vi "arduino_data_and_filters_subIV.vi"(7 "loop iteration number":i32, 8 "arduino 1-6 address and errors":T3, 11 "arduinos on?":bool) -> (0 "arduino 1-6 addresses and errors out":T2, 1 "arduino 1-6 data out":T1, 3 "arduinos on? output":bool)   [LabVIEW 2014]
uses:
  LabVIEW QCM code version 4 Working/(SubVI)2 2QCM.vi
  LabVIEW QCM code version 4 Working/(SubVI)1 3QCM.vi
  LabVIEW QCM code version 4 Working/(SubVI)2 3QCM.vi
  LabVIEW QCM code version 4 Working/(SubVI)1 4QCM.vi
  LabVIEW QCM code version 4 Working/(SubVI)2 4QCM.vi
  LabVIEW QCM code version 4 Working/(SubVI)1 5QCM.vi
  LabVIEW QCM code version 4 Working/(SubVI)2 5QCM.vi
  LabVIEW QCM code version 4 Working/(SubVI)1 6QCM.vi
  LabVIEW QCM code version 4 Working/(SubVI)2 6QCM.vi
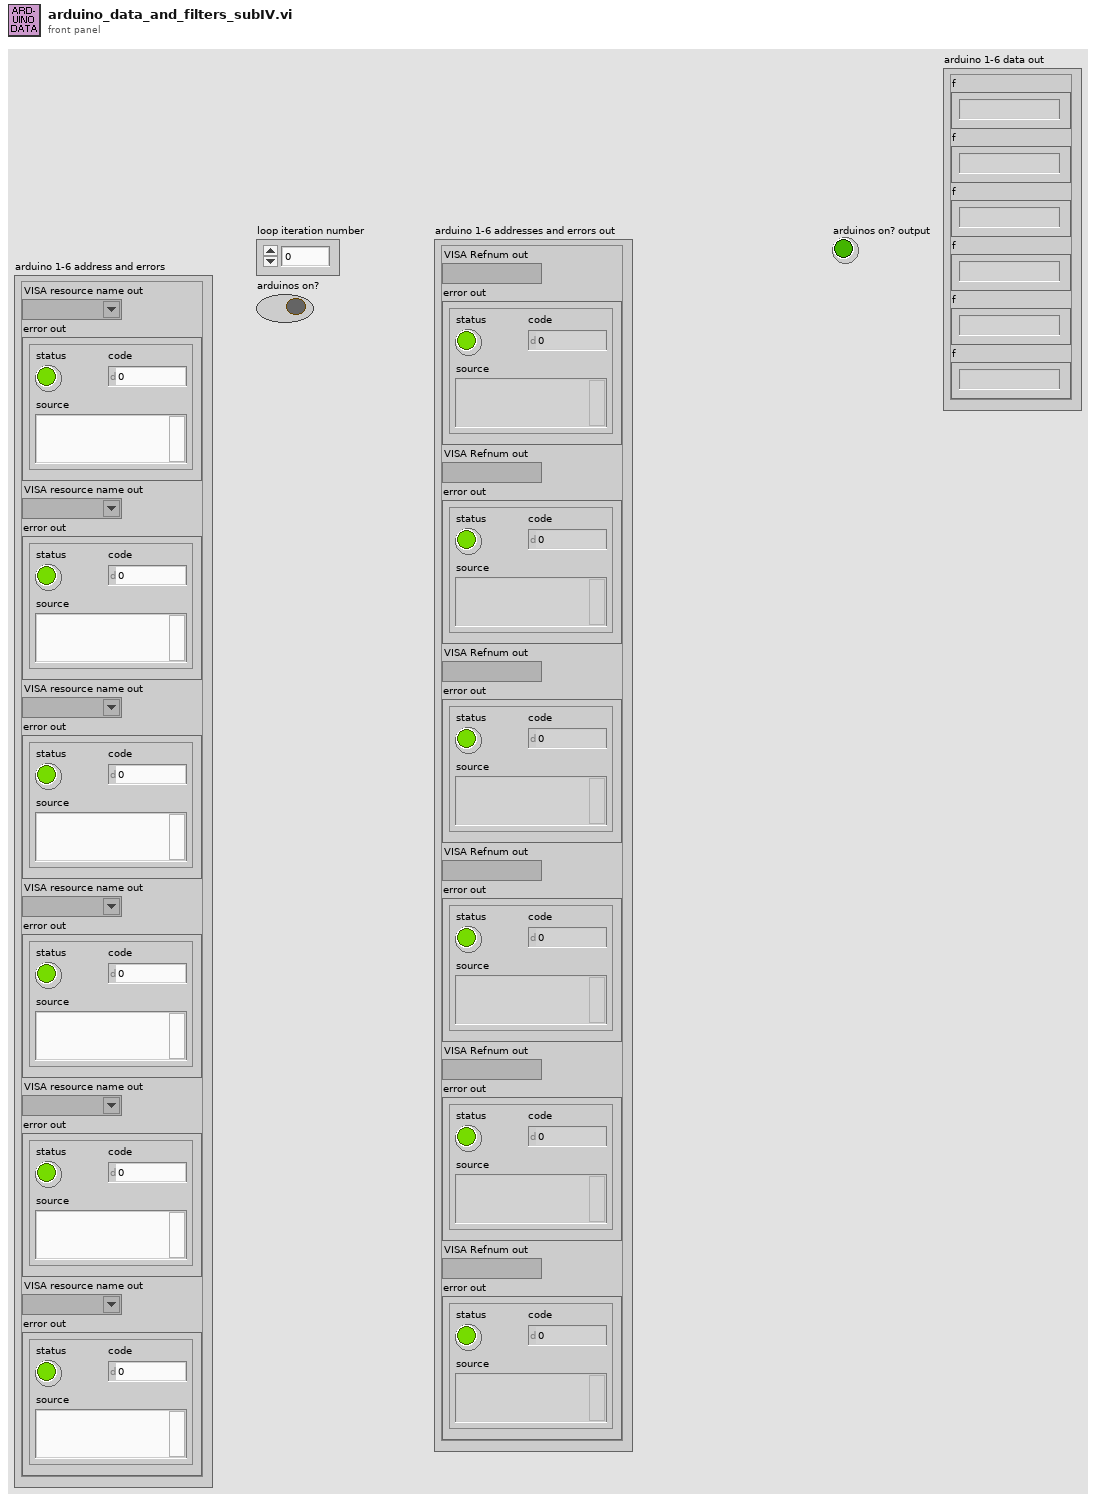
[diagram p1: front panel]
types:
  T1 = cluster{"f":string, "f":string, "f":string, "f":string, "f":string, "f":string}
  T2 = cluster{"VISA Refnum out":refnum<visa-resource-name>, "error out":errorcluster, "VISA Refnum out":refnum<visa-resource-name>, "error out":errorcluster, "VISA Refnum out":refnum<visa-resource-name>, "error out":errorcluster, "VISA Refnum out":refnum<visa-resource-name>, "error out":errorcluster, "VISA Refnum out":refnum<visa-resource-name>, "error out":errorcluster, "VISA Refnum out":refnum<visa-resource-name>, "error out":errorcluster}
  T3 = cluster{"VISA resource name out":refnum<visa-resource-name>, "error out":errorcluster, "VISA resource name out":refnum<visa-resource-name>, "error out":errorcluster, "VISA resource name out":refnum<visa-resource-name>, "error out":errorcluster, "VISA resource name out":refnum<visa-resource-name>, "error out":errorcluster, "VISA resource name out":refnum<visa-resource-name>, "error out":errorcluster, "VISA resource name out":refnum<visa-resource-name>, "error out":errorcluster}
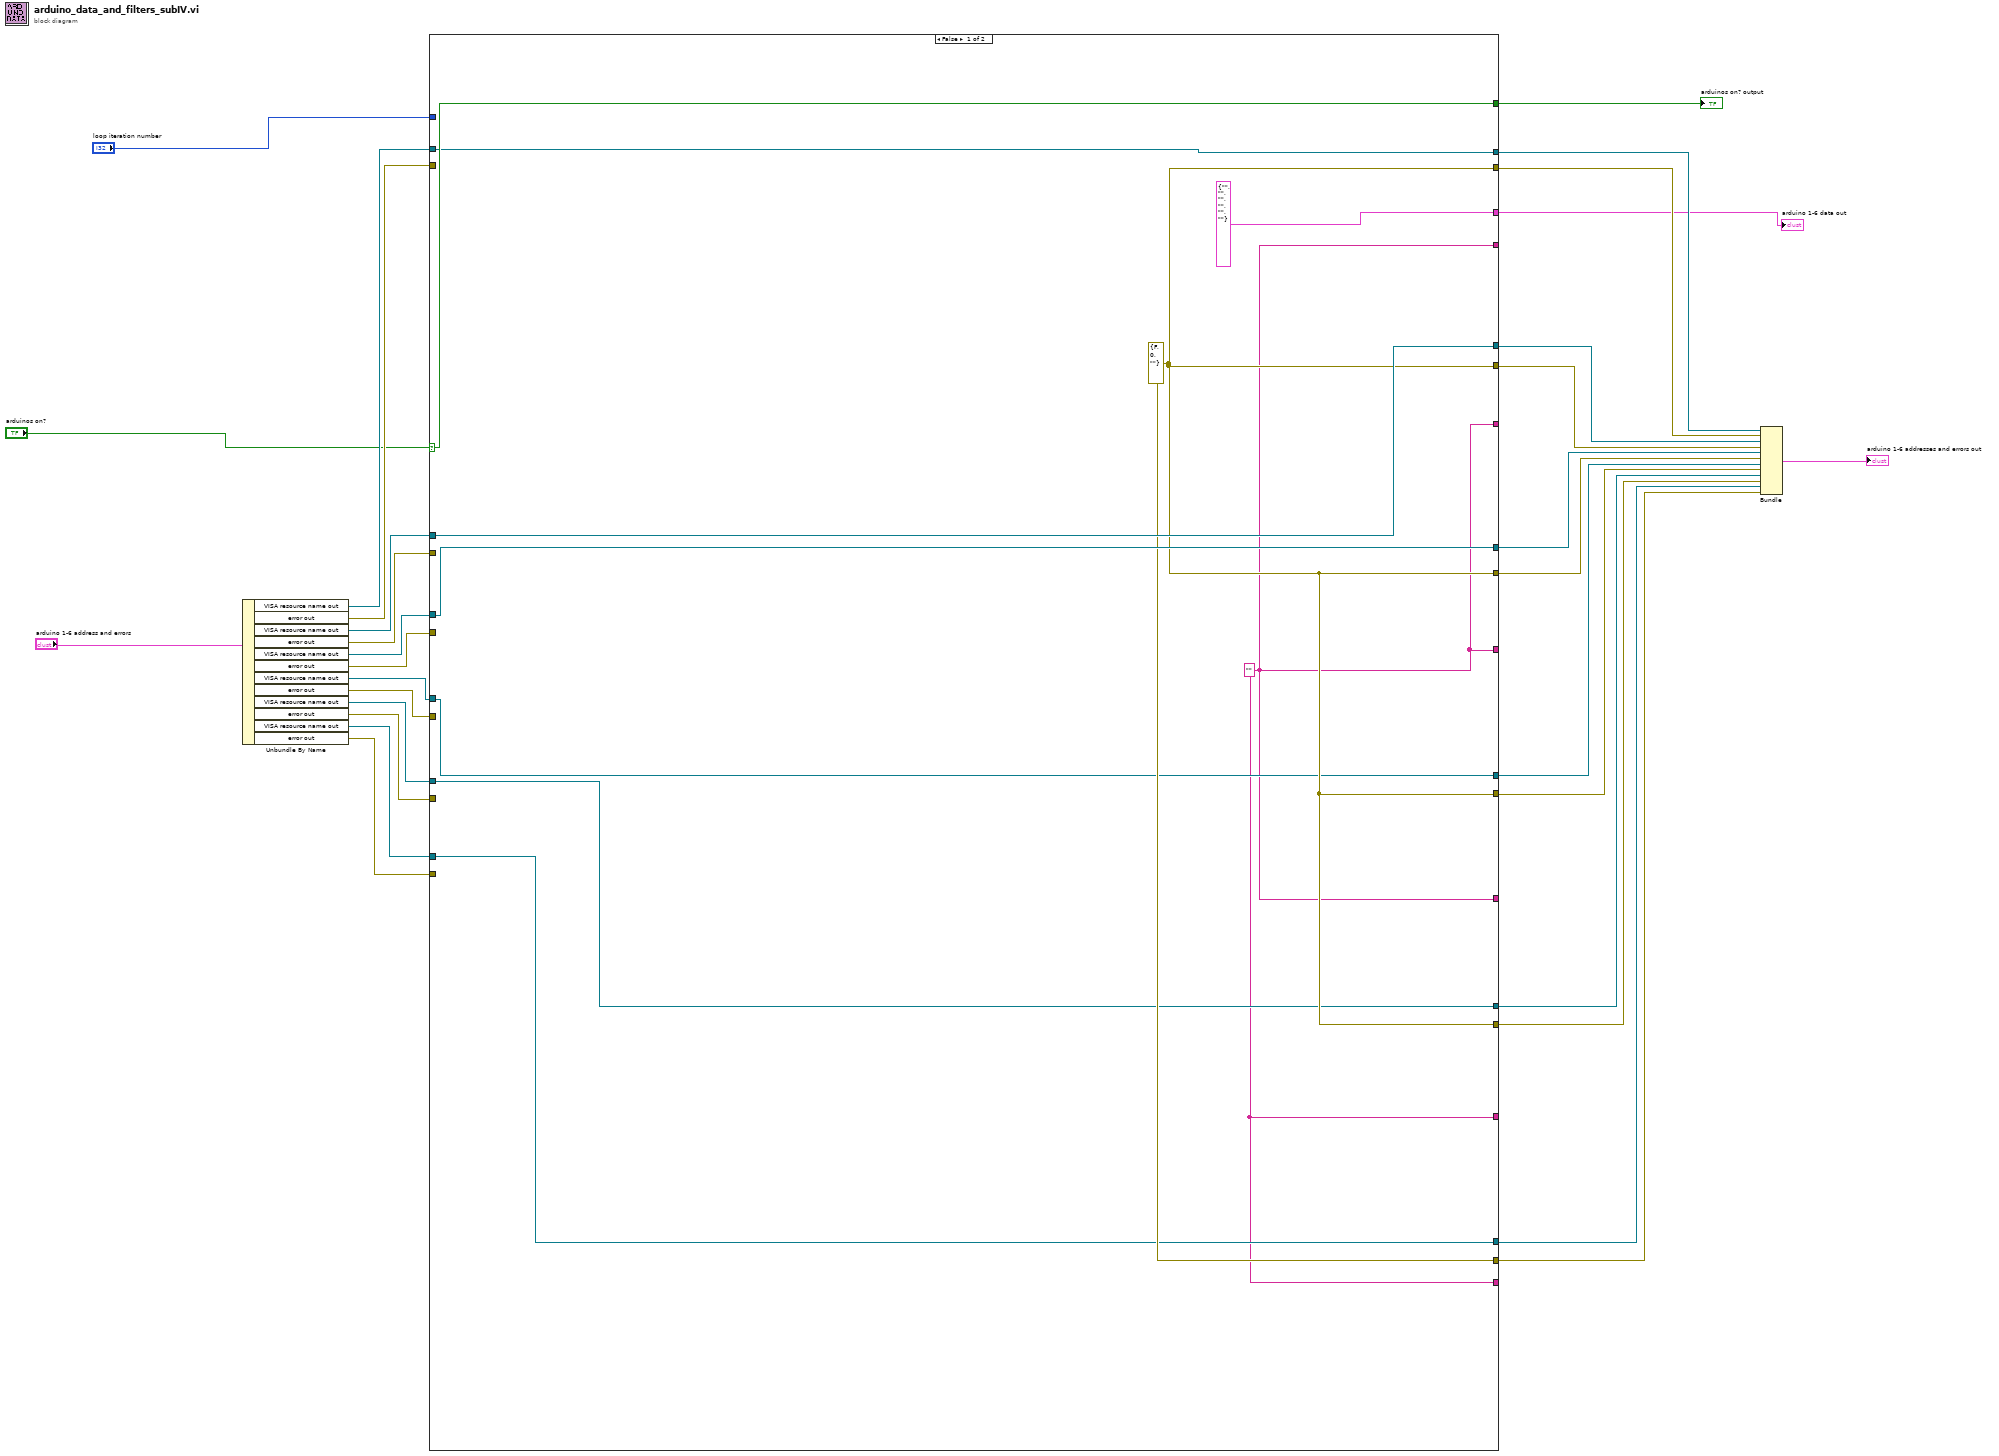
[diagram p0: block diagram]
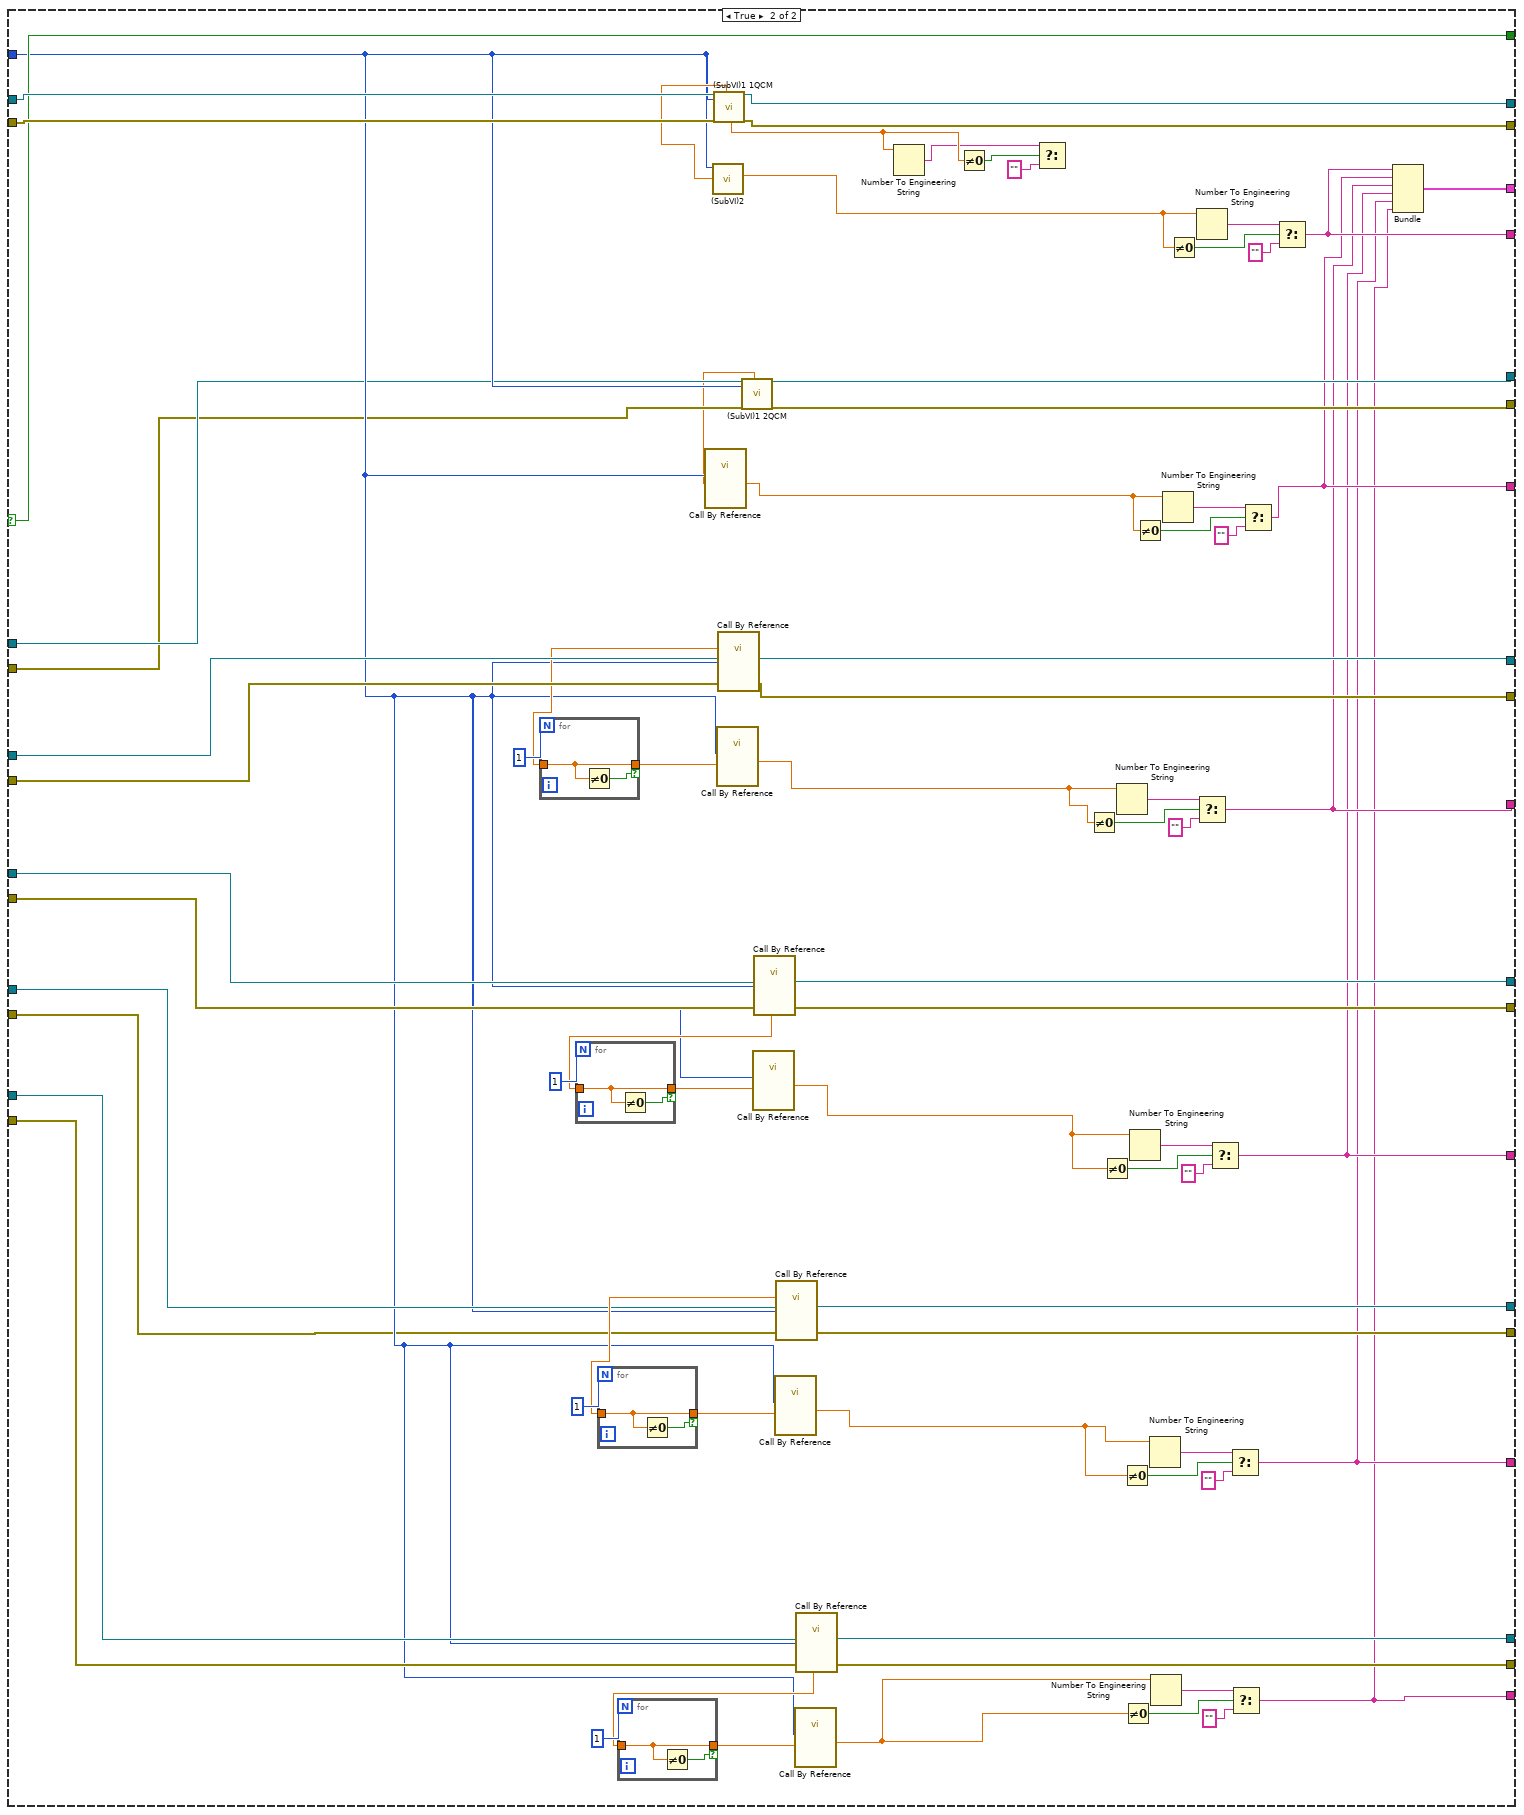
[diagram p2: hidden frame]
diagram:
  n1 = Unbundle By Name("arduino 1-6 address and errors") -> ("VISA resource name out"=w29:refnum<visa-resource-name>, "error out"=w27:errorcluster, "VISA resource name out"=w26:refnum<visa-resource-name>, "error out"=w25:errorcluster, "VISA resource name out"=w24:refnum<visa-resource-name>, "error out"=w23:errorcluster, "VISA resource name out"=w22:refnum<visa-resource-name>, "error out"=w21:errorcluster, "VISA resource name out"=w20:refnum<visa-resource-name>, "error out"=w19:errorcluster, "VISA resource name out"=w18:refnum<visa-resource-name>, "error out"=w17:errorcluster)
  n2 = case shown="False" "arduinos on?" {
    selector: "arduinos on?" -> [w40 w84]
    tunnel: [w40 w84] -> w2
    tunnel: w29 -> [w39 w107]
    tunnel: w27 -> [_ w108]
    tunnel: [w36 w106] -> w14
    tunnel: [w39 w105] -> w15
    tunnel: "loop iteration number" -> [_ w54]
    tunnel: w26 -> [w38 w53]
    tunnel: w25 -> [_ w50]
    tunnel: [w38 w52] -> w13
    tunnel: [w36 w51] -> w12
    tunnel: w24 -> [w37 w113]
    tunnel: w23 -> [_ w112]
    tunnel: [w37 w110] -> w11
    tunnel: [w36 w109] -> w10
    tunnel: w22 -> [w35 w95]
    tunnel: w21 -> [_ w94]
    tunnel: w20 -> [w34 w93]
    tunnel: w19 -> [_ w48]
    tunnel: w18 -> [w33 w91]
    tunnel: w17 -> [_ w92]
    tunnel: [w36 w90] -> w8
    tunnel: [w35 w89] -> w9
    tunnel: [w34 w88] -> w7
    tunnel: [w36 w87] -> w6
    tunnel: [w33 w86] -> w5
    tunnel: [w36 w85] -> w4
    tunnel: [w32 w47] -> _
    tunnel: [w32 w46] -> _
    tunnel: [w32 w45] -> _
    tunnel: [w32 w42] -> _
    tunnel: [w32 w43] -> _
    tunnel: [w32 w44] -> _
    tunnel: [T1 {"f"="", "f"="", "f"="", "f"="", "f"="", "f"=""} w41] -> w1
    frame False {
      w32 = "" ("f")
      w36 = errorcluster {"status"=FALSE, "code"=0, "source"=""} ("error out")
    }
    frame True {
      n3 = call "(SubVI)1 1QCM.vi"("VISA Refnum in"=w107, "main loop iteration number"=w54, "error in (no error)"=w108) -> ("Freq out"=w55:dbl, "unfiltered freq out"=w83:dbl, "VISA Refnum out"=w105:refnum<visa-resource-name>, "error out"=w106:errorcluster)  [unwired: 11 in, 2 out]
      n4 = call "(SubVI)2.vi"("Freq in"=w55, "loop iteration number"=w54) -> ("Mean"=w76:dbl)  [unwired: 6 in, 3 out]
      n5 = call-by-ref "?"("VISA Refnum in"=w113, "Numeric in"=w54, "error in (no error)"=w112) -> ("Numeric out"=w111:dbl, "VISA Refnum out"=w110:refnum<visa-resource-name>, "error out"=w109:errorcluster)  [unwired: 7 in, 11 out]
      n6 = for {
        N: 1 -> [_]
        tunnel: w111 -> [w123]
        tunnel: [w123] -> w115 if=w122
        n7 = Not Equal To 0?(x=w123) -> (x != 0?=w122:bool)
      }
      n8 = call-by-ref "?"("Numeric in"=w115, "Numeric"=w54) -> ("Mean"=w68:dbl)  [unwired: 8 in, 5 out]
      n9 = call "(SubVI)1 2QCM.vi"("VISA Refnum in"=w53, "Numeric in"=w54, "error in (no error)"=w50) -> ("Numeric out"=w49:dbl, "VISA Refnum out"=w52:refnum<visa-resource-name>, "error out"=w51:errorcluster)  [unwired: 5 in, 9 out]
      n10 = call-by-ref "?"("Numeric in"=w49, "Numeric"=w54) -> ("Mean"=w72:dbl)  [unwired: 8 in, 5 out]
      n11 = call-by-ref "?"("VISA Refnum in"=w95, "Numeric in"=w54, "error in (no error)"=w94) -> ("Numeric out"=w102:dbl, "VISA Refnum out"=w89:refnum<visa-resource-name>, "error out"=w90:errorcluster)  [unwired: 7 in, 11 out]
      n12 = for {
        N: 1 -> [_]
        tunnel: w102 -> [w121]
        tunnel: [w121] -> w104 if=w120
        n13 = Not Equal To 0?(x=w121) -> (x != 0?=w120:bool)
      }
      n14 = call-by-ref "?"("Numeric in"=w104, "Numeric"=w54) -> ("Mean"=w56:dbl)  [unwired: 8 in, 5 out]
      n15 = call-by-ref "?"("VISA Refnum in"=w93, "Numeric in"=w54, "error in (no error)"=w48) -> ("Numeric out"=w99:dbl, "VISA Refnum out"=w88:refnum<visa-resource-name>, "error out"=w87:errorcluster)  [unwired: 7 in, 11 out]
      n16 = for {
        N: 1 -> [_]
        tunnel: w99 -> [w119]
        tunnel: [w119] -> w101 if=w118
        n17 = Not Equal To 0?(x=w119) -> (x != 0?=w118:bool)
      }
      n18 = call-by-ref "?"("Numeric in"=w101, "Numeric"=w54) -> ("Mean"=w57:dbl)  [unwired: 8 in, 5 out]
      n19 = call-by-ref "?"("VISA Refnum in"=w91, "Numeric in"=w54, "error in (no error)"=w92) -> ("Numeric out"=w96:dbl, "VISA Refnum out"=w86:refnum<visa-resource-name>, "error out"=w85:errorcluster)  [unwired: 7 in, 11 out]
      n20 = for {
        N: 1 -> [_]
        tunnel: w96 -> [w117]
        tunnel: [w117] -> w98 if=w116
        n21 = Not Equal To 0?(x=w117) -> (x != 0?=w116:bool)
      }
      n22 = call-by-ref "?"("Numeric in"=w98, "Numeric"=w54) -> ("Mean"=w58:dbl)  [unwired: 8 in, 5 out]
      n23 = Number To Engineering String(4:w83) -> (0:w81:string)  [unwired: 3 in]
      n24 = Not Equal To 0?(x=w83) -> (x != 0?=w82:bool)
      n25 = Select(t=w81, s=w82, f="") -> ()  [unwired: 1 out]
      n26 = Not Equal To 0?(x=w68) -> (x != 0?=w71:bool)
      n27 = Not Equal To 0?(x=w56) -> (x != 0?=w65:bool)
      n28 = Number To Engineering String(4:w68) -> (0:w70:string)  [unwired: 3 in]
      n29 = Not Equal To 0?(x=w57) -> (x != 0?=w64:bool)
      n30 = Not Equal To 0?(x=w58) -> (x != 0?=w59:bool)
      n31 = Number To Engineering String(4:w56) -> (0:w66:string)  [unwired: 3 in]
      n32 = Not Equal To 0?(x=w72) -> (x != 0?=w73:bool)
      n33 = Number To Engineering String(4:w57) -> (0:w63:string)  [unwired: 3 in]
      n34 = Number To Engineering String(4:w58) -> (0:w60:string)  [unwired: 3 in]
      n35 = Number To Engineering String(4:w72) -> (0:w74:string)  [unwired: 3 in]
      n36 = Not Equal To 0?(x=w76) -> (x != 0?=w77:bool)
      n37 = Number To Engineering String(4:w76) -> (0:w78:string)  [unwired: 3 in]
      n38 = Select(t=w70, s=w71, f="") -> (s? t:f=w45:string)
      n39 = Select(t=w66, s=w65, f="") -> (s? t:f=w44:string)
      n40 = Select(t=w63, s=w64, f="") -> (s? t:f=w43:string)
      n41 = Select(t=w60, s=w59, f="") -> (s? t:f=w42:string)
      n42 = Select(t=w74, s=w73, f="") -> (s? t:f=w46:string)
      n43 = Select(t=w78, s=w77, f="") -> (s? t:f=w47:string)
      n44 = Bundle("f"=w47, "f"=w46, "f"=w45, "f"=w44, "f"=w43, "f"=w42) -> (w41:T1)  [unwired: 1 in]
    }
  }
  "arduinos on? output" <- w2
  "arduino 1-6 data out" <- w1
  n45 = Bundle("VISA Refnum out"=w15, "error out"=w14, "VISA Refnum out"=w13, "error out"=w12, "VISA Refnum out"=w11, "error out"=w10, "VISA Refnum out"=w9, "error out"=w8, "VISA Refnum out"=w7, "error out"=w6, "VISA Refnum out"=w5, "error out"=w4) -> (→"arduino 1-6 addresses and errors out":T2)  [unwired: 1 in]
